vi "Common PS Boolean to UINT8.vi"(8 "error in (no error)":errorcluster, 10 "PS ON-OFF":bool[](array[boolean]), 11 "Inverse PS Matrix Mapping":u32[][](array[numeric])) -> (0 "error out":errorcluster, 3 "PS ON-OFF (per PS Rack)":u8[](array[numeric]))   [LabVIEW 2011, in "Common VIs.lvlib"]
doc: "Encode the digital I/O of all Actuation Chassis from a vector of boolean values to a byte representation grouped by Actuation chassis."
uses:
  Common VIs.lvlib
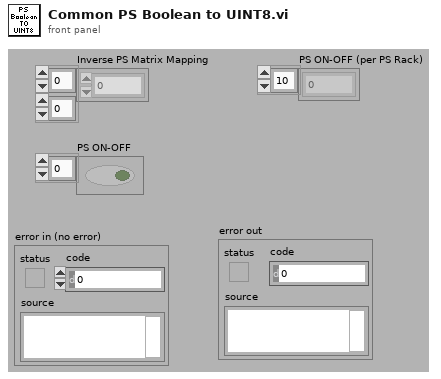
[diagram p1: front panel]
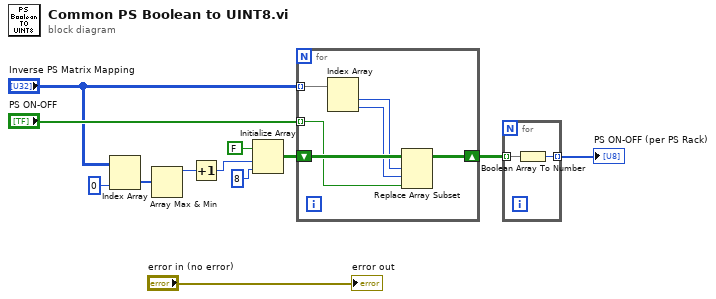
[diagram p0: block diagram]
diagram:
  n1 = Index Array(array="Inverse PS Matrix Mapping", index (col)=0 ("disabled index (col)")) -> (element=w4:u32[])  [unwired: 1 in]
  n2 = Array Max & Min(array=w4) -> (max value=w6:u32)  [unwired: 3 out]
  n3 = Increment(x=w6) -> (x+1=w2:u32)
  n4 = Initialize Array(FALSE, w2, 8 ("dimension size")) -> (w9:bool[][])
  n5 = for {
    tunnel: "PS ON-OFF" -> [w14] mode=indexing
    tunnel: "Inverse PS Matrix Mapping" -> [w17] mode=indexing
    shift-right: [w13] -> w11
    shift-left: w9 -> [w18]
    n6 = Index Array(array=w17) -> (element #1=w16:u32, element #2=w15:u32)  [unwired: 2 in]
    n7 = Replace Array Subset(array=w18, new element=w14, index (row)=w16, index (col)=w15) -> (w13:bool[][])
  }
  n8 = for {
    tunnel: w11 -> [w20] mode=indexing
    tunnel: [w19] -> w12 mode=indexing
    n9 = Boolean Array To Number(Boolean array=w20) -> (number=w19:u8)
  }
  "PS ON-OFF (per PS Rack)" <- w12
  "error out" <- "error in (no error)"
